vi "JKI With AMC.vi"   [LabVIEW 2017]
uses:
  GPower/String/GPString.lvlib
types:
  T1 = enum16{"Any", "Alphanumeric", "Binary", "Hexadecimal", "Letters", "Lower case", "Numbers", "Octal", "Printable", "Upper case"}
  T2 = typedef "amc_Message Queue.ctl" = refnum<queue>
  T3 = enum32{"Invalid", "Standard", "Closed", "Hidden", "Minimized", "Maximized"}
  T4 = enum32{"invalid app kind", "Development System", "Run Time System", "Student Edition", "Embedded LabVIEW", "Evaluation", "Custom"}
  T5 = cluster{"Core":cluster{"Current VI Reference":refnum<vi>, "Close Panel on Exit?":bool}, "Your Boolean data":bool, "Your string data":string}
  T6 = cluster{"Current VI Reference":refnum<vi>, "Close Panel on Exit?":bool}
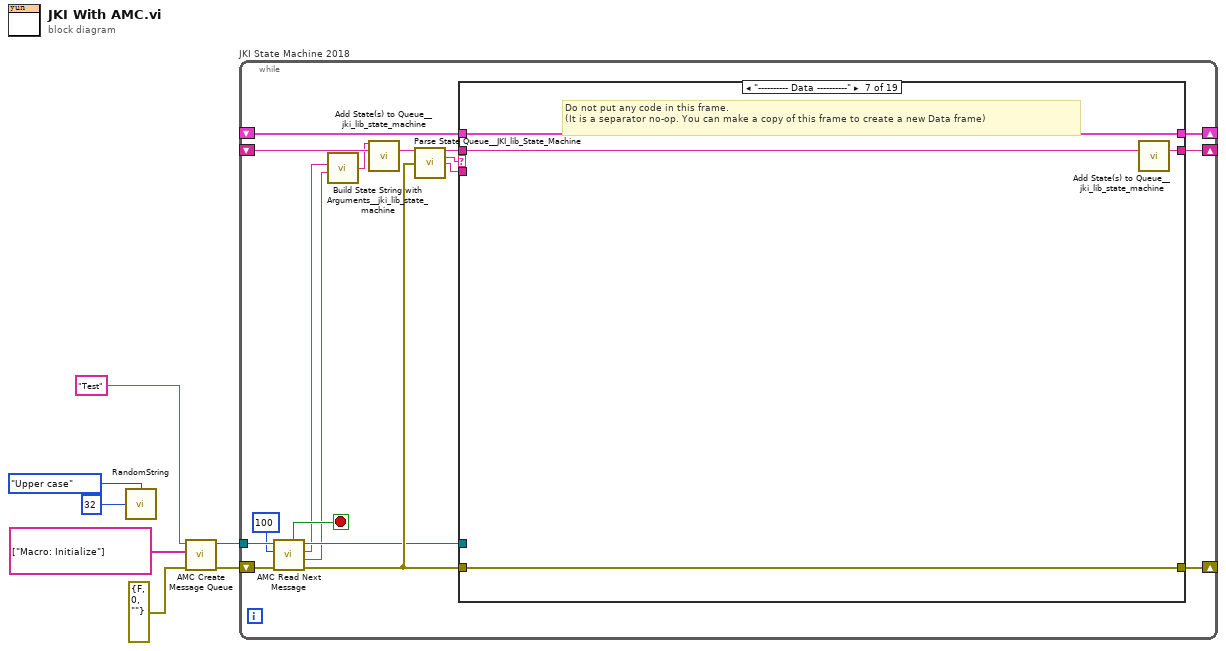
[diagram p0: block diagram]
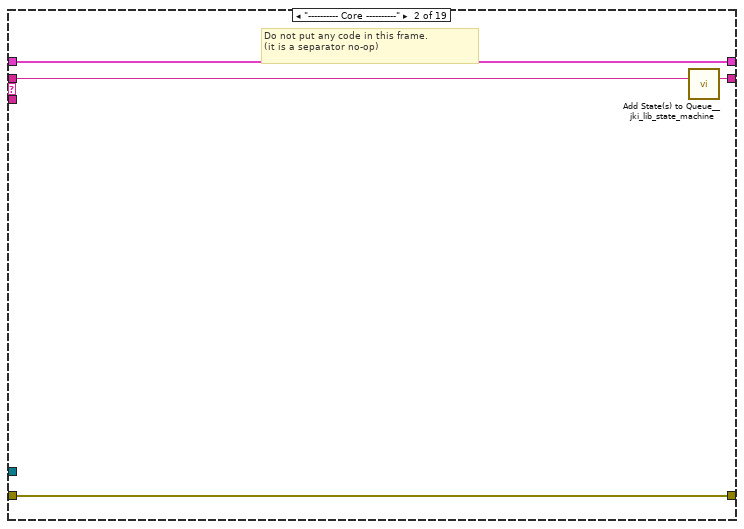
[diagram p3: hidden frame]
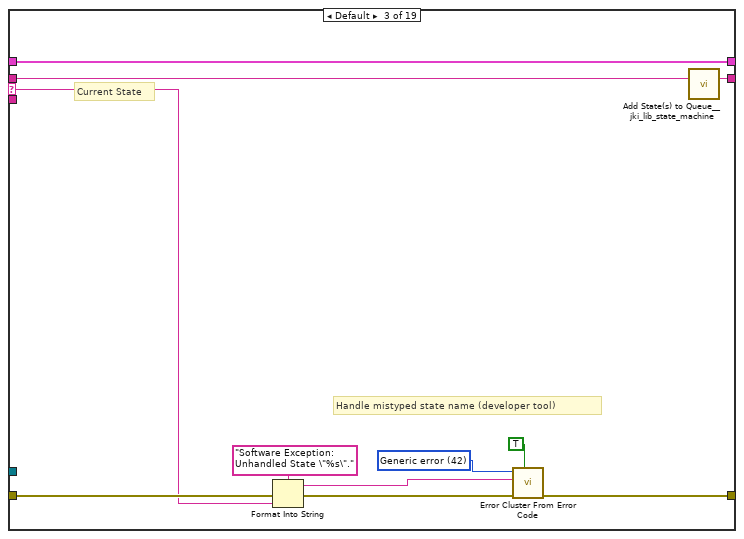
[diagram p4: hidden frame]
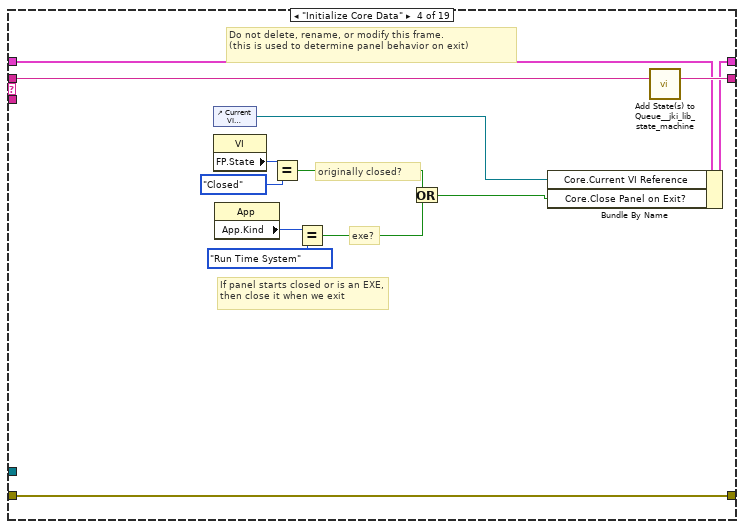
[diagram p5: hidden frame]
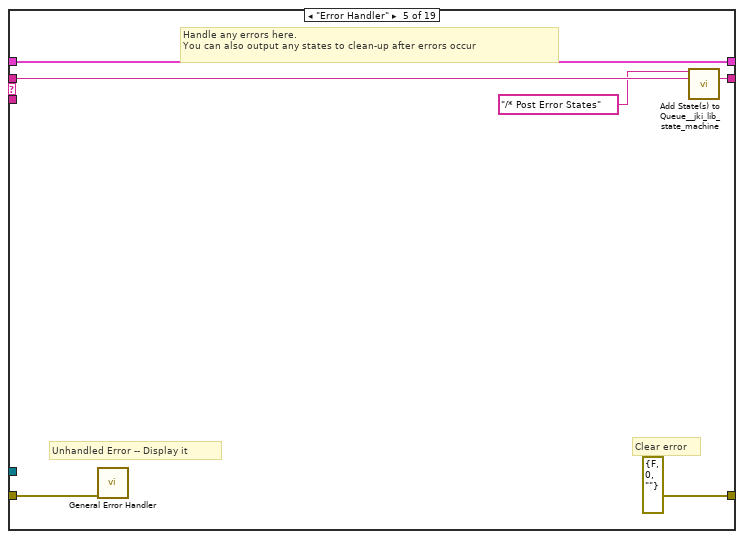
[diagram p6: hidden frame]
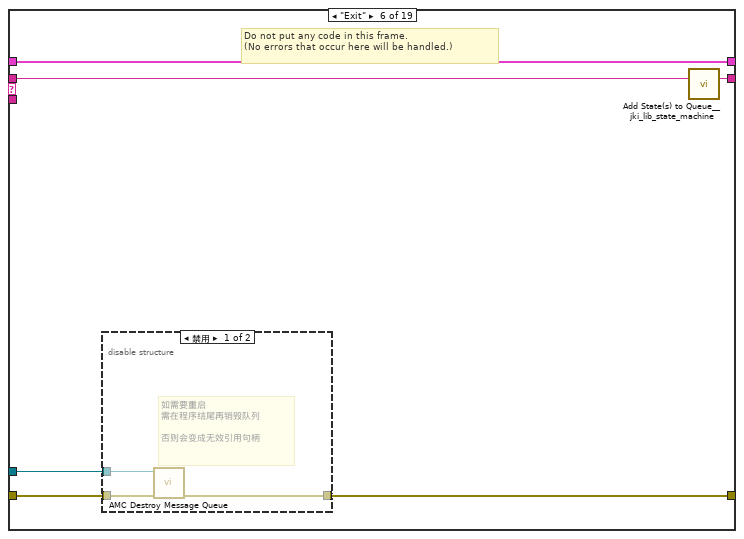
[diagram p7: hidden frame]
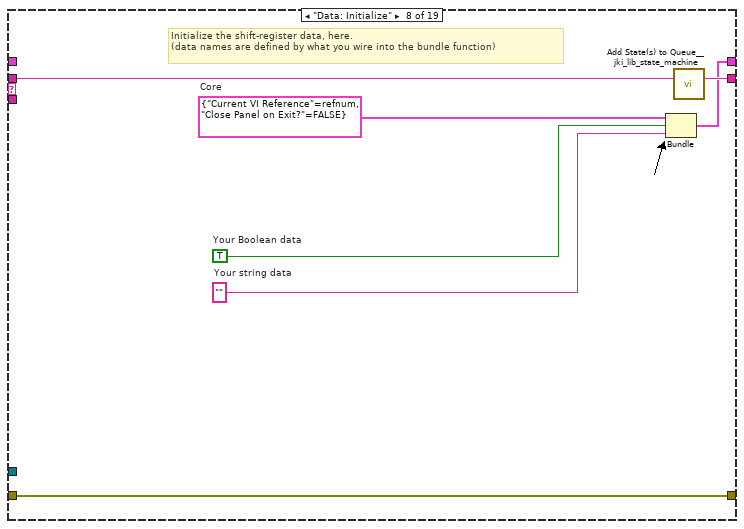
[diagram p9: hidden frame]
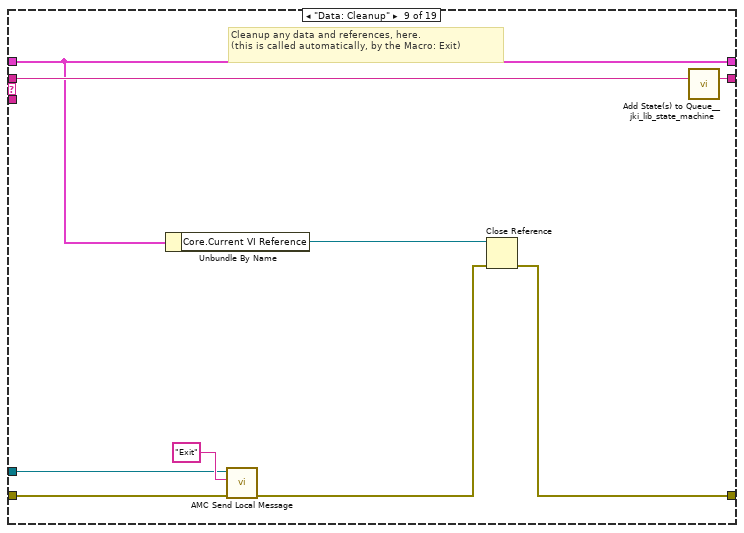
[diagram p10: hidden frame]
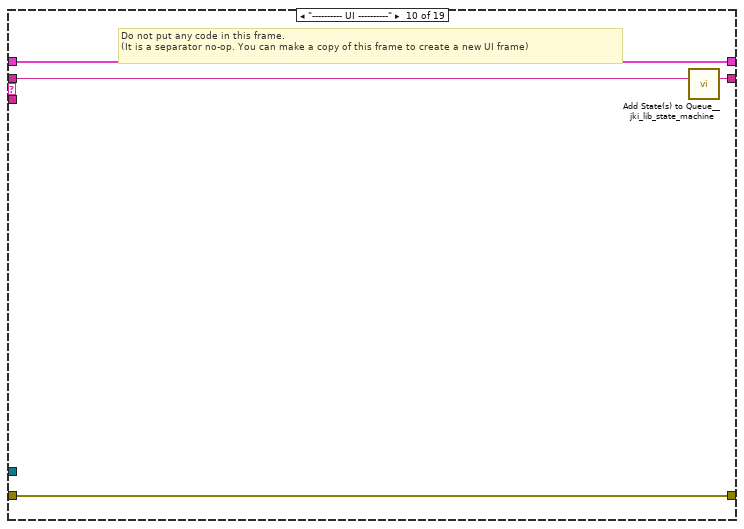
[diagram p11: hidden frame]
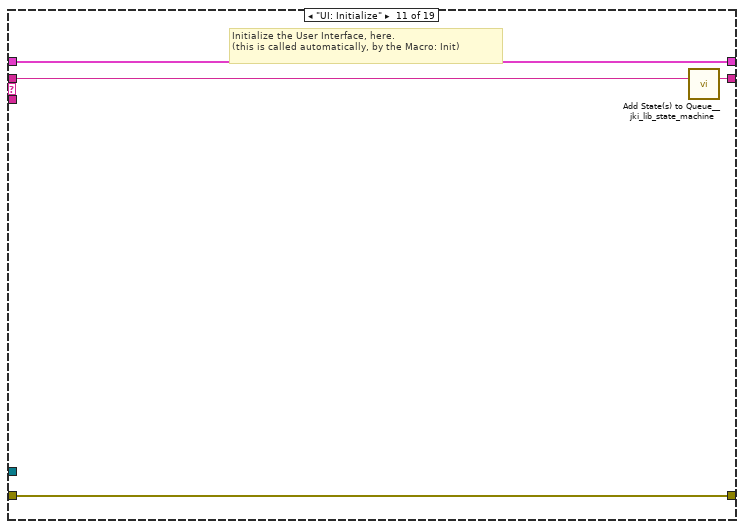
[diagram p12: hidden frame]
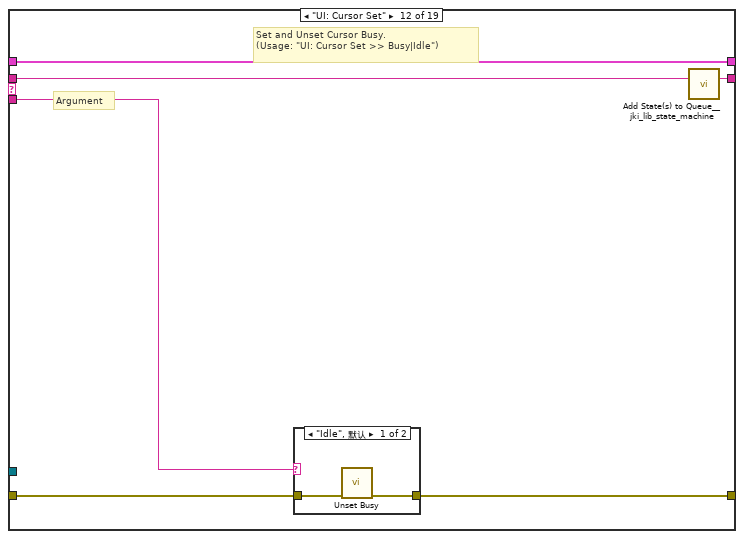
[diagram p13: hidden frame]
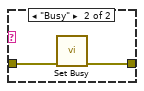
[diagram p14: hidden frame]
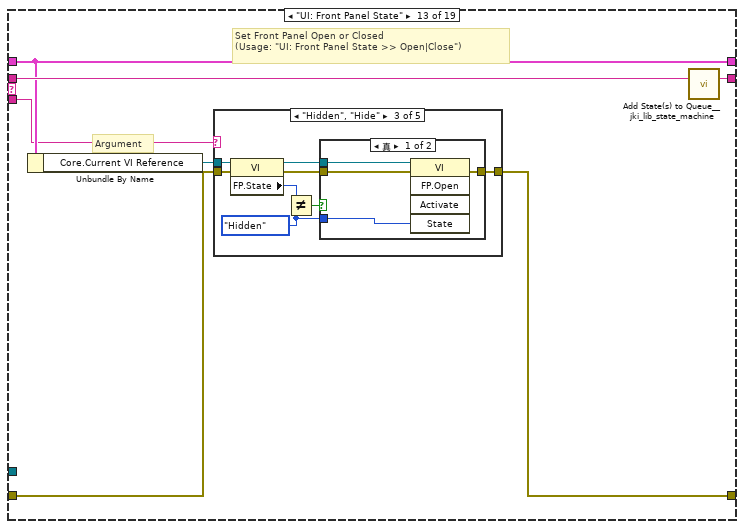
[diagram p15: hidden frame]
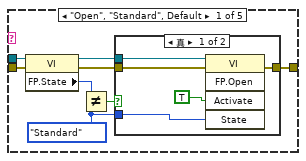
[diagram p16: hidden frame]
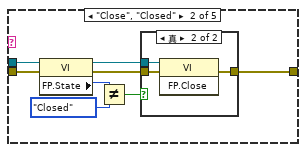
[diagram p18: hidden frame]
diagram:
  n1 = call "RandomString.vi"("Randomness"=32, "Allowed characters"=T1."Upper case") -> ()  [unwired: 1 out]
  n2 = call "AMC Create Message Queue.vi"("error in (no error)"=errorcluster {"status"=FALSE, "code"=0, "source"=""}, "Initial Message Names"=string[] ["Macro: Initialize"], "Message Queue Name"="Test") -> ("error out"=w6:errorcluster, "Message Queue out"=w3:T2)  [unwired: 7 in]
  n3 = while "JKI State Machine 2018" {
    shift-right: [w20] -> _
    shift-left: _ -> [w19]
    shift-right: [w22] -> _
    shift-left: w6 -> [w18]
    shift-right: [w21] -> _
    shift-left: _ -> [w12]
    tunnel: w3 -> [w16]
    stop <- w13 stop-if-true
    n4 = call "AMC Read Next Message.vi"("error in (no error)"=w18, "timeout (1ms)"=100, "Message Queue in"=w16) -> ("error out"=w17:errorcluster, "Message Value"=w9:string, "Message Name"=w10:string, "Message Queue out"=w15:T2, "Exit Process"=w13:bool)  [unwired: 1 in, 3 out]
    n5 = call "Build State String with Arguments__jki_lib_state_machine.vi"("Arguments (\"\")"=w9, "State"=w10) -> ("State with Arguments"=w8:string)  [unwired: 4 in]
    n6 = call "Add State(s) to Queue__jki_lib_state_machine.vi"("State(s) in Front (\"\")"=w8, "State(s) in (\"\")"=w12) -> ("States Out"=w11:string)  [unwired: 13 in]
    n7 = call "Parse State Queue__JKI_lib_State_Machine.vi"("State Queue"=w11, "Error In (no error)"=w17) -> ("Remaining States"=w24:string, "Current State"=w25:string, "Arguments"=w23:string)  [unwired: 10 in, 1 out]
    n8 = case shown="\"---------- Data ----------\"" w25 {
      selector: w25 -> [_ _ w33 _ _ _ _ _ _ _ _ _ _ _ _ _ _ _ _]
      tunnel: w24 -> [w27 w32 w37 w56 w62 w68 w76 w83 w92 w96 w100 w106 w117 w186 w191 w201 w205 w210 w214]
      tunnel: w23 -> [_ _ _ _ _ _ _ _ _ _ _ w101 w111 _ _ _ _ w206 _]
      tunnel: w19 -> [w28 w29 w35 w49 w59 w66 w73 _ w86 w93 w98 w104 w113 w183 w188 w199 w202 w207 w211]
      tunnel: [w26 w30 w39 w53 errorcluster {"status"=FALSE, "code"=0, "source"=""} ("error out") w63 w74 w80 w84 w94 w97 w102 w114 w184 w189 w192 w203 w208 w212] -> w22
      tunnel: w17 -> [w26 w30 w38 w53 w58 w64 w74 w80 w88 w94 w97 w103 w115 w184 w189 w192 w203 w208 w212]
      tunnel: [w27 w31 w36 w55 w61 w67 w75 w82 w91 w95 w99 w105 w116 w185 w190 w200 w204 w209 w213] -> w21
      tunnel: [w28 w29 w35 w54 w59 w66 w73 w81 w86 w93 w98 w104 w113 w183 w188 w199 w202 w207 w211] -> w20
      tunnel: w15 -> [_ _ _ _ _ w65 _ _ w89 _ _ _ _ _ _ _ _ _ _]
      frame "", "Event Structure", "Idle" {
      }
      frame "---------- Core ----------" {
        # "Do not put any code in this frame.\n(it is a separator no-op)"
        n9 = call "Add State(s) to Queue__jki_lib_state_machine.vi"("State(s) in (\"\")"=w32) -> ("States Out"=w31:string)  [unwired: 14 in]
      }
      frame Default {
        w42 = 42 items=["No error", "Argument error", "Memory is full", "Out of zone", "End of file", "File already open", "Generic file I/O error", "File not found", "File permission error", "Disk is full", "Duplicate path", "Too many files open", "System feature not enabled", "Resource file not found", "Cannot add resource", "Resource not found", "Image not found", "Image memory error", "Pen does not exist", "Config type invalid", "Config token not found", "Config parse error", "Config memory error", "Bad external code format", "Bad external code offset", "External code not present", "Null window", "Destroy window error", "Null menu", "Print aborted", "Bad print record", "Print driver error", "Windows error during printing", "Memory error during printing", "Print dialog error", "Generic print error", "Invalid device refnum", "Device not found", "Device parameter error", "Device unit error", "Cannot open device", "Device call aborted", "Generic error", "Cancelled by user", "Object ID too low", "Object ID too high", "Object not in heap", "Unknown heap", "Unknown object (invalid DefProc)", "Unknown object (DefProc not in table)", "Message out of range", "Invalid (null) method", "Unknown message", "Manager call not supported", "Bad address", "Network operation in progress", "Network operation timed out", "Connection is busy", "Network attribute not supported", "Network error", "Address in use", "System out of memory", "Connection aborted", "Connection refused", "Not connected", "Already connected", "Connection closed", "Initialization error (interapplication manager)", "Bad occurrence", "Wait on unbound occurrence handler", "Occurrence queue overflow", "Datalog type conflict", "Unused", "Unrecognized type (interapplication manager)", "Memory corrupt", "Failed to make temporary DLL", "Old CIN version", "Drag socket not found", "Failed to load drop-object", "Failed to register OLE object", "Failed to release OLE object", "Format specifier type mismatch", "Unknown format specifier", "Too few format specifiers", "Too many format specifiers", "Scan failed", "Newer CIN version", "Error converting to variant", "Runtime menu error", "Password tampered", "Variant attribute not found", "Incompatible variant data type", "Event data is not available", "Event Store is not present", "Occurrence is not found", "Event Queue is not created", "Event info is not available", "Refnum passed is NULL", "Error retrieving Class GUID", "Error retrieving CoClass GUID", "Error retrieving TypeLib GUID.", "Bad built application magic bytes.", "Specific driver is different from the specific driver associated with the Logical Name.", "There is no session opened to the class driver.", "Max Error", "MAX - Error with config objects", "MAX - Error loading configuration", "MAX - Group not supported"]
        # "Current State"
        # "Handle mistyped state name (developer tool)"
        n10 = Format Into String(format string="Software Exception: Unhandled State \"%s\"." ("message"), error in=w38, w33) -> (resulting string=w41:string, error out=w40:errorcluster)  [unwired: 1 in]
        n11 = call <vilib>:"Error Cluster From Error Code.vi"("show call chain? (False)"=TRUE, "error in (no error)"=w40, "error message (\"\")"=w41, "error code (0)"=w42) -> ("error out"=w39:errorcluster)  [unwired: 5 in]
        n12 = call "Add State(s) to Queue__jki_lib_state_machine.vi"("State(s) in (\"\")"=w37) -> ("States Out"=w36:string)  [unwired: 14 in]
      }
      frame "Initialize Core Data" {
        # "Do not delete, rename, or modify this frame.\n(this is used to determine panel behavior on exit)"
        # "originally closed?"
        # "exe?"
        # "If panel starts closed or is an EXE, then close it when we exit"
        n13 = control-ref of="Current VI Reference"() -> (w47:refnum<vi>)
        n14 = property class="VI"() -> ("FP.State"=w46:T3)  [unwired: 2 in, 2 out]
        n15 = property class="App"() -> ("App.Kind"=w52:T4)  [unwired: 2 in, 2 out]
        n16 = Equal?(x=w46, y=T3."Closed" ("Front Panel Window:State")) -> (x = y?=w44:bool)
        n17 = Equal?(x=w52, y=T4."Run Time System" ("Application:Kind")) -> (x = y?=w50:bool)
        n18 = Or(x=w44, y=w50) -> (x .or. y?=w48:bool)
        n19 = Bundle By Name(cluster=w49, "Core.Current VI Reference"=w47, "Core.Close Panel on Exit?"=w48) -> (w54:T5)
        n20 = call "Add State(s) to Queue__jki_lib_state_machine.vi"("State(s) in (\"\")"=w56) -> ("States Out"=w55:string)  [unwired: 14 in]
      }
      frame "Error Handler" {
        # "Unhandled Error -- Display it"
        # "Handle any errors here.\nYou can also output any states to clean-up after errors occur"
        # "Clear error"
        n21 = call <vilib>:"General Error Handler.vi"("error in (no error)"=w58) -> ()  [unwired: 10 in, 5 out]
        n22 = call "Add State(s) to Queue__jki_lib_state_machine.vi"("State(s) in Front (\"\")"="/* Post Error States", "State(s) in (\"\")"=w62) -> ("States Out"=w61:string)  [unwired: 13 in]
      }
      frame "Exit" {
        # "Do not put any code in this frame.\n(No errors that occur here will be handled.)"
        n23 = disable-structure shown="禁用" {
          disable-tunnel: w65 -> [w71 _]
          disable-tunnel: w64 -> [w70 w72]
          disable-tunnel: [w69 w72] -> w63
          frame Disabled {
            # "如需要重启\n需在程序结尾再销毁队列\n\n否则会变成无效引用句柄"
            n24 = call "AMC Destroy Message Queue.vi"("error in (no error)"=w70, "Message Queue in"=w71) -> ("error out"=w69:errorcluster)  [unwired: 9 out]
          }
          frame Enabled {
          }
        }
        n25 = call "Add State(s) to Queue__jki_lib_state_machine.vi"("State(s) in (\"\")"=w68) -> ("States Out"=w67:string)  [unwired: 14 in]
      }
      frame "---------- Data ----------" {
        # "Do not put any code in this frame.\n(It is a separator no-op. You can make a copy of this frame to create a new Data frame)"
        n26 = call "Add State(s) to Queue__jki_lib_state_machine.vi"("State(s) in (\"\")"=w76) -> ("States Out"=w75:string)  [unwired: 14 in]
      }
      frame "Data: Initialize" {
        w77 = T6 {"Current VI Reference"=refnum, "Close Panel on Exit?"=FALSE}  # Core
        w79 = TRUE  # Your Boolean data
        w78 = ""  # Your string data
        # "Initialize the shift-register data, here.\n(data names are defined by what you wire into the bundle function)"
        n27 = Bundle("Core"=w77, "Your Boolean data"=w79, "Your string data"=w78) -> (w81:T5)  [unwired: 1 in]
        n28 = call "Add State(s) to Queue__jki_lib_state_machine.vi"("State(s) in (\"\")"=w83) -> ("States Out"=w82:string)  [unwired: 14 in]
      }
      frame "Data: Cleanup" {
        # "Cleanup any data and references, here.\n(this is called automatically, by the Macro: Exit)"
        n29 = Unbundle By Name(w86) -> ("Core.Current VI Reference"=w87:refnum<vi>)
        n30 = call "AMC Send Local Message.vi"("error in (no error)"=w88, "Message Name"="Exit", "Message Queue in"=w89) -> ("error out"=w85:errorcluster)  [unwired: 7 in, 1 out]
        n31 = Close Reference(reference=w87, error in (no error)=w85) -> (error out=w84:errorcluster)
        n32 = call "Add State(s) to Queue__jki_lib_state_machine.vi"("State(s) in (\"\")"=w92) -> ("States Out"=w91:string)  [unwired: 14 in]
      }
      frame "---------- UI ----------" {
        # "Do not put any code in this frame.\n(It is a separator no-op. You can make a copy of this frame to create a new UI frame)"
        n33 = call "Add State(s) to Queue__jki_lib_state_machine.vi"("State(s) in (\"\")"=w96) -> ("States Out"=w95:string)  [unwired: 14 in]
      }
      frame "UI: Initialize" {
        # "Initialize the User Interface, here.\n(this is called automatically, by the Macro: Init)"
        n34 = call "Add State(s) to Queue__jki_lib_state_machine.vi"("State(s) in (\"\")"=w100) -> ("States Out"=w99:string)  [unwired: 14 in]
      }
      frame "UI: Cursor Set" {
        # "Argument"
        # "Set and Unset Cursor Busy.\n(Usage: \"UI: Cursor Set >> Busy|Idle\")"
        n35 = case shown="\"Idle\", 默认" w101 {
          tunnel: w103 -> [w108 w110]
          tunnel: [w107 w109] -> w102
          frame "Idle", Default {
            n36 = call <vilib>:"Unset Busy.vi"("error in (no error)"=w108) -> ("error out"=w107:errorcluster)  [unwired: 10 in]
          }
          frame "Busy" {
            n37 = call <vilib>:"Set Busy.vi"("error in (no error)"=w110) -> ("error out"=w109:errorcluster)  [unwired: 9 in, 1 out]
          }
        }
        n38 = call "Add State(s) to Queue__jki_lib_state_machine.vi"("State(s) in (\"\")"=w106) -> ("States Out"=w105:string)  [unwired: 14 in]
      }
      frame "UI: Front Panel State" {
        # "Argument"
        # "Set Front Panel Open or Closed\n(Usage: \"UI: Front Panel State >> Open|Close\")"
        n39 = Unbundle By Name(w113) -> ("Core.Current VI Reference"=w112:refnum<vi>)
        n40 = case shown="\"Hidden\", \"Hide\"" w111 {
          tunnel: w115 -> [w123 w138 w149 w162 w175]
          tunnel: [w125 w139 w151 w164 w177] -> w114
          tunnel: w112 -> [w124 w136 w150 w163 w176]
          frame "Open", "Standard", Default {
            w118 = T3."Standard" ("State")
            n41 = property class="VI"(reference=w124, error in=w123) -> (reference out=w121:refnum<vi>, error out=w122:errorcluster, "FP.State"=w120:T3)
            n42 = Not Equal?(x=w120, y=w118) -> (x != y?=w119:bool)
            n43 = case shown="真" w119 {
              tunnel: [w129 w131] -> w125
              tunnel: w122 -> [w128 w131]
              tunnel: w121 -> [w127 _]
              tunnel: w118 -> [w126 _]
              frame True {
                n44 = invoke class="VI" method="FP.Open"(reference=w127, error in=w128, "Activate"=TRUE, "State"=w126) -> (error out=w129:errorcluster)  [unwired: 1 in, 4 out]
              }
              frame False {
              }
            }
          }
          frame "Close", "Closed" {
            n45 = property class="VI"(reference=w136, error in=w138) -> (reference out=w135:refnum<vi>, error out=w137:errorcluster, "FP.State"=w133:T3)
            n46 = Not Equal?(x=w133, y=T3."Closed" ("Front Panel Window:State")) -> (x != y?=w132:bool)
            n47 = case shown="真" w132 {
              tunnel: [w140 w143] -> w139
              tunnel: w137 -> [w140 w142]
              tunnel: w135 -> [_ w141]
              frame False {
              }
              frame True {
                n48 = invoke class="VI" method="FP.Close"(reference=w141, error in=w142) -> (error out=w143:errorcluster)  [unwired: 1 in, 2 out]
              }
            }
          }
          frame "Hidden", "Hide" {
            w144 = T3."Hidden" ("State")
            n49 = property class="VI"(reference=w150, error in=w149) -> (reference out=w147:refnum<vi>, error out=w148:errorcluster, "FP.State"=w146:T3)
            n50 = Not Equal?(x=w146, y=w144) -> (x != y?=w145:bool)
            n51 = case shown="真" w145 {
              tunnel: [w155 w156] -> w151
              tunnel: w148 -> [w154 w156]
              tunnel: w147 -> [w153 _]
              tunnel: w144 -> [w152 _]
              frame True {
                n52 = invoke class="VI" method="FP.Open"(reference=w153, error in=w154, "State"=w152) -> (error out=w155:errorcluster)  [unwired: 2 in, 4 out]
              }
              frame False {
              }
            }
          }
          frame "Minimize", "Minimized" {
            w157 = T3."Minimized" ("State")
            n53 = property class="VI"(reference=w163, error in=w162) -> (reference out=w160:refnum<vi>, error out=w161:errorcluster, "FP.State"=w159:T3)
            n54 = Not Equal?(x=w159, y=w157) -> (x != y?=w158:bool)
            n55 = case shown="真" w158 {
              tunnel: [w168 w169] -> w164
              tunnel: w161 -> [w167 w169]
              tunnel: w160 -> [w166 _]
              tunnel: w157 -> [w165 _]
              frame True {
                n56 = invoke class="VI" method="FP.Open"(reference=w166, error in=w167, "State"=w165) -> (error out=w168:errorcluster)  [unwired: 2 in, 4 out]
              }
              frame False {
              }
            }
          }
          frame "Maximize", "Maximized" {
            w170 = T3."Maximized" ("State")
            n57 = property class="VI"(reference=w176, error in=w175) -> (reference out=w173:refnum<vi>, error out=w174:errorcluster, "FP.State"=w172:T3)
            n58 = Not Equal?(x=w172, y=w170) -> (x != y?=w171:bool)
            n59 = case shown="真" w171 {
              tunnel: [w181 w182] -> w177
              tunnel: w174 -> [w180 w182]
              tunnel: w173 -> [w179 _]
              tunnel: w170 -> [w178 _]
              frame True {
                n60 = invoke class="VI" method="FP.Open"(reference=w179, error in=w180, "State"=w178) -> (error out=w181:errorcluster)  [unwired: 2 in, 4 out]
              }
              frame False {
              }
            }
          }
        }
        n61 = call "Add State(s) to Queue__jki_lib_state_machine.vi"("State(s) in (\"\")"=w117) -> ("States Out"=w116:string)  [unwired: 14 in]
      }
      frame "---------- Macro ----------" {
        # "Do not put any code in this frame.\n(It is a separator no-op. You can make a copy of this frame to create a new Macro frame)"
        n62 = call "Add State(s) to Queue__jki_lib_state_machine.vi"("State(s) in (\"\")"=w186) -> ("States Out"=w185:string)  [unwired: 14 in]
      }
      frame "Macro: Initialize" {
        w187 = "Data: Initialize\nInitialize Core Data\nUI: Initialize\nUI: Front Panel State >> Hidden"  # Data: Initialize Initialize Core Data UI: Initialize UI: Front Panel State >> Hidden
        # "Initialization Macro\n(This is called once, when the VI starts)"
        n63 = call "Add State(s) to Queue__jki_lib_state_machine.vi"("State(s) in Front (\"\")"=w187, "State(s) in (\"\")"=w191) -> ("States Out"=w190:string)  [unwired: 13 in]
      }
      frame "Macro: Exit" {
        # "Exit Macro\n(This is called once, when the VI exits)"
        n64 = Unbundle By Name(w199) -> ("Core.Close Panel on Exit?"=w198:bool)
        n65 = Select(t="UI: Front Panel State >> Close", s=w198, f="") -> (s? t:f=w195:string)
        n66 = call "Add State(s) to Queue__jki_lib_state_machine.vi"("State(s) in (\"\")"=w195, "State(s) at Back (\"\")"="Data: Cleanup\nExit") -> ("States Out"=w193:string)  [unwired: 13 in]
        n67 = call "Add State(s) to Queue__jki_lib_state_machine.vi"("State(s) in Front (\"\")"=w193, "State(s) in (\"\")"=w201) -> ("States Out"=w200:string)  [unwired: 13 in]
      }
      frame "---------- New Category ----------" {
        n68 = call "Add State(s) to Queue__jki_lib_state_machine.vi"("State(s) in (\"\")"=w205) -> ("States Out"=w204:string)  [unwired: 14 in]
      }
      frame "Test" {
        n69 = One Button Dialog(message=w206) -> ()  [unwired: 1 in, 1 out]
        n70 = call "Add State(s) to Queue__jki_lib_state_machine.vi"("State(s) in (\"\")"=w210) -> ("States Out"=w209:string)  [unwired: 14 in]
      }
      frame "New Category: 2" {
        # "Your code here.\n(You can make a copy of, or modify, this frame)"
        n71 = call "Add State(s) to Queue__jki_lib_state_machine.vi"("State(s) in (\"\")"=w214) -> ("States Out"=w213:string)  [unwired: 14 in]
      }
    }
  }
